vi "Simulator Tool Loop Dialog.vi"(1 "Tool Sim W1":u16, 2 "Tool Sim  W2":u16, 11 "error in (no error)":errorcluster) -> ()   [LabVIEW 2011]
uses:
  Measurments Handling/Status Digitalish.ctl
  Measurments Handling/Common/Variable List Common Analog.ctl
  Tool/Variable List Tool Analog.ctl
  Measurments Handling/Common/Variable List Common Digital.ctl
  Tool/Variable List Tool Digital.ctl
  Modem Status/Variable List Modem Status Analog.ctl
  Modem Status/Variable List Modem Status Digital.ctl
  Tool simulator data.ctl
  emi Lib/System 01/0 - General/App/Loop control 2/Private/_emi_SMLoop Control Single.vi
  emi Lib/System 01/0 - General/App/Loop control 2/Private/_emi_ SMLoop start condition.vi
  emi Lib/System 01/0 - General/App/Loop control 2/Private/_emi_ SMLoop Error Check.vi
  emi Lib/Basic/0 - General/Error/emi_Is Error.vi
  emi Lib/System 01/0 - General/App/Loop control 2/Private/_emi_SMLoop Register new.vi
  emi Lib/System 01/0 - General/S&E reporting/emi_Send S&E Error message.vi
  emi Lib/Basic/0 - General/Error/emi_ Is Error state.vi
  emi Lib/System 01/0 - General/emi_Read System ID.vi
  emi Lib/System 01/0 - General/App/Loop control/Private/_emi_GFV Loop Running.vi
  emi Lib/System 01/0 - General/App/Loop control 2/Private/_emi_ SMLoop Restart Counter.vi
  emi Lib/System 01/0 - General/App/Loop control/Private/_emi_GFV stop a loop so it can reset.vi
  emi Lib/System 01/0 - General/App/Loop control 2/Private/_emi_ SMLoop Restart.vi
  emi Lib/System 01/0 - General/App/Loop control/Private/_emi_GFV Loop Linking.vi
  emi Lib/System 01/0 - General/App/Loop control/Private/_emi_GFV Loop Enable.vi
  emi Lib/System 01/0 - General/App/Private/_emi_GFV App Close.vi
  emi Lib/System 01/0 - General/Private/_emi_GFV System ID.vi
  emi Lib/System 01/0 - General/S&E reporting/Private/_emi_S&E Q Generator.vi
  <vilib>/Utility/VariantDataType/GetNumericInfo.vi
  emi Lib/System 01/0 - General/Debug/Private/_emi_GFV Debug Disp.vi
panel:
  in  "Modem Status Digital Data":cluster{"Channel Name":string, "Status in":T1}[](array[cluster])
  in  "Modem Status Analog Data":T2(array[cluster]) {"Value" scale=0.0..100.0}
  in  "Tool Digital Data":cluster{"Channel Name":string, "Status in":T1}[](array[cluster])
  in  "PCP Digital Data":cluster{"Channel Name":string, "Status in":T1}[](array[cluster])
  in  "Loop timer - increase to create timeout":u32=250
  in  "PCP Simulator Data":T2(array[cluster]) {"Value" scale=0.0..100.0}
  in  "Simulator Data":T2(array[cluster]) {"Value" scale=0.0..200.0}
  # "Modem Status Data"
  # "PCP Data"
  # "Limited Tool simulator for GUI testing.\n\nNOTE: No tool behavior or properties should be infered absed on this simulator\ncapability. All tool capability and propertied information should go via propper\nproject channels."
  # "TOOL DATA"
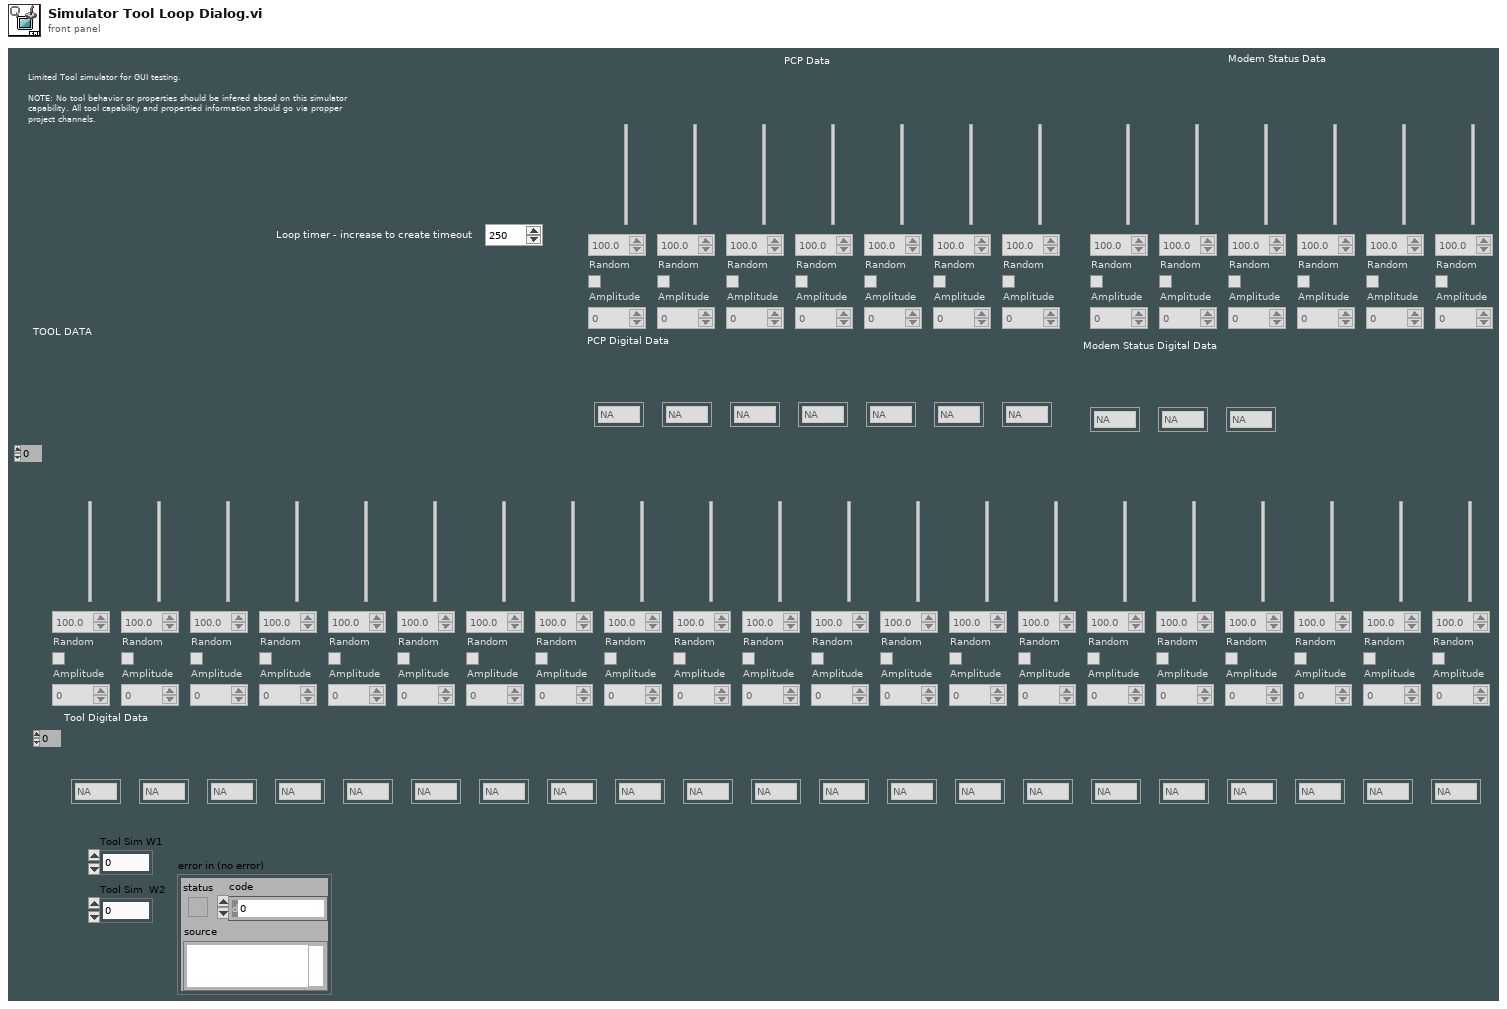
[diagram p1: front panel]
types:
  T1 = typedef "Status Digitalish.ctl" = enum16{"NA", "False", "True"}
  T2 = cluster{"Channel Name":string, "Value":dbl, "Random":bool, "Amplitude":dbl}[]
  T3 = typedef "Variable List Modem Status Digital.ctl" = enum16{"TMU_LINK_STATUS"}
  T4 = typedef "Variable List Modem Status Analog.ctl" = enum16{"TS_Signal_Quality", "TS_PCB_Temp", "TS_Gain", "DH_Signal_Quality", "DH_PCB_Temp", "DH_Gain", "Link_Status"}
  T5 = cluster{"Channel Name":string, "Value":dbl, "Random":bool, "Amplitude":dbl}
  T6 = typedef "Variable List Tool Digital.ctl" = enum16{"Tool Error Controller", "Tool Stopped Controller", "Tool Relay 1", "Tool Relay 2", "Tool Both Relays", "Tool node Pressure 1", "Tool Error Pressure 1", "Tool Stopped Pressure 1", "Tool node Pressure 2", "Tool Error Pressure 2", "Tool Stopped Pressure 2", "Tool node Solenoid", "Tool Error Solenoid", "Tool Stopped Solenoid", "Tool Solenoid 1", "Tool Solenoid 2", "Tool Solenoid 3", "Tool node PSU", "Tool Error PSU", "Tool Stopped PSU", "Upper Tension Sub", "Tool Error Upper Tension Sub", "Tool Stopped Upper Tension Sub", "Lower Tension Sub", "Tool Error Lower Tension Sub", "Tool Stopped Lower Tension Sub", "Stroke Target seeking", "Stroke Moving Out", "Stroke Moving Inn", "Stroke valves set for Out", "Stroke valves set for In", "Stroke In (force)", "Stroke Out (force)", "Stroke Force decreasing(in)", "Stroke Force decreasing(out)", "Stroke Force change not correct", "Stroke SLIPS established P1", "Stroke SLIPS established P2", "Stroke SLIPS established", "Stroke Pressure Monitor Ongoing", "Stroke Pressure Monitor Ending ", "Tool Stroke enable Valve", "Tool Stroke direction Valve", "Tool Anchor Valve", "Stroker Var19 - Reserved", "Stroker Var20 - Reserved", "Stroker Var21 - Reserved", "Stroker Var22 - Reserved", "Stroker Var23 - Reserved", "Stroker Var24 - Reserved", "Tractor Var1 - Reserved", "Tractor Var2 - Reserved", "Tractor Var3 - Reserved", "Tractor Var4 - Reserved", "Tractor Var5 - Reserved", "Tractor Var6 - Reserved", "Tractor Var7 - Reserved", "Tractor Var8 - Reserved", "Oil filling mode", "Mill Bit Direction", "Position control", "Anchor", "Driller Var5 - Reserved", "Driller Var6 - Reserved", "Driller Var7 - Reserved", "Driller Var8 - Reserved"}
  T7 = typedef "Variable List Common Digital.ctl" = enum16{"PCP Connected", "PCP PC Control", "HV PSU connected", "HV PSU HV Active", "Modem Connected", "Tool Connected", "CanBus interface"}
  T8 = typedef "Variable List Tool Analog.ctl" = enum16{"Tool Max Temperature", "Tool (Controller) Temperature", "Tool Supply Voltage", "Tool (Controller) Current", "Tool Acceleration X", "Tool Acceleration Y", "Tool Acceleration Z", "Tool Acceleration Sum", "Tool Inclination", "Tool Rotation", "Tool GP Sensor 1", "Tool GP Sensor 2", "Tool (Pressure 1) Temperature", "Tool Pressure 1 RAW", "Tool (Pressure 2) Temperature", "Tool Pressure 2 RAW", "Tool (Solenoid) Temperature", "Tool Solenoid Position", "PSU Temp", "Head Voltage", "PSU Main Voltage out", "PSU Main Current out", "Upper Tension Sub Temp", "Tool Upper Tension Sub Raw", "Lower Tension Sub Temp", "Tool Lower Tension Sub Raw", "Tool Var27 - Reserved", "Tool Var28 - Reserved", "Tool Var29 - Reserved", "Tool Var30 - Reserved", "Stroke Extension", "Stroke In Force", "Stroke Out Force", "Stroke Force", "Stroker Pressure 1", "Stroker Pressure 2", "Stroker Upper Tension Sub", "Stroker Lower Tension Sub", "Stroker Var09 - Reserved", "Stroker Var10 - Reserved", "Tractor Upper Tension Sub", "Tractor Lower Tension Sub", "Tractor Var03 - Reserved", "Tractor Var04 - Reserved", "Tool Temperature sensor", "Tool Motor Voltage", "Tool Motor Current", "Tool Motor Torque", "Tool weight on bit", "Tool Motor RPM"}
  T9 = typedef "Variable List Common Analog.ctl" = enum16{"HVPSU Head Voltage", "HVPSU TS Voltage", "HVPSU Current", "PCP Cable Resistance", "Winch Depth", "Winch Line Speed", "Winch Wire Tension"}
  T10 = typedef "Tool simulator data.ctl" = cluster{"Analog Values":dbl[], "Digital Values":T1[]}
  T11 = typedef "_emi_ SMLoop sates.ctl" = enum16{"Init", "Standby", "Start", "Normal Operation", "Stop", "Error Handling", "End", "Post"}
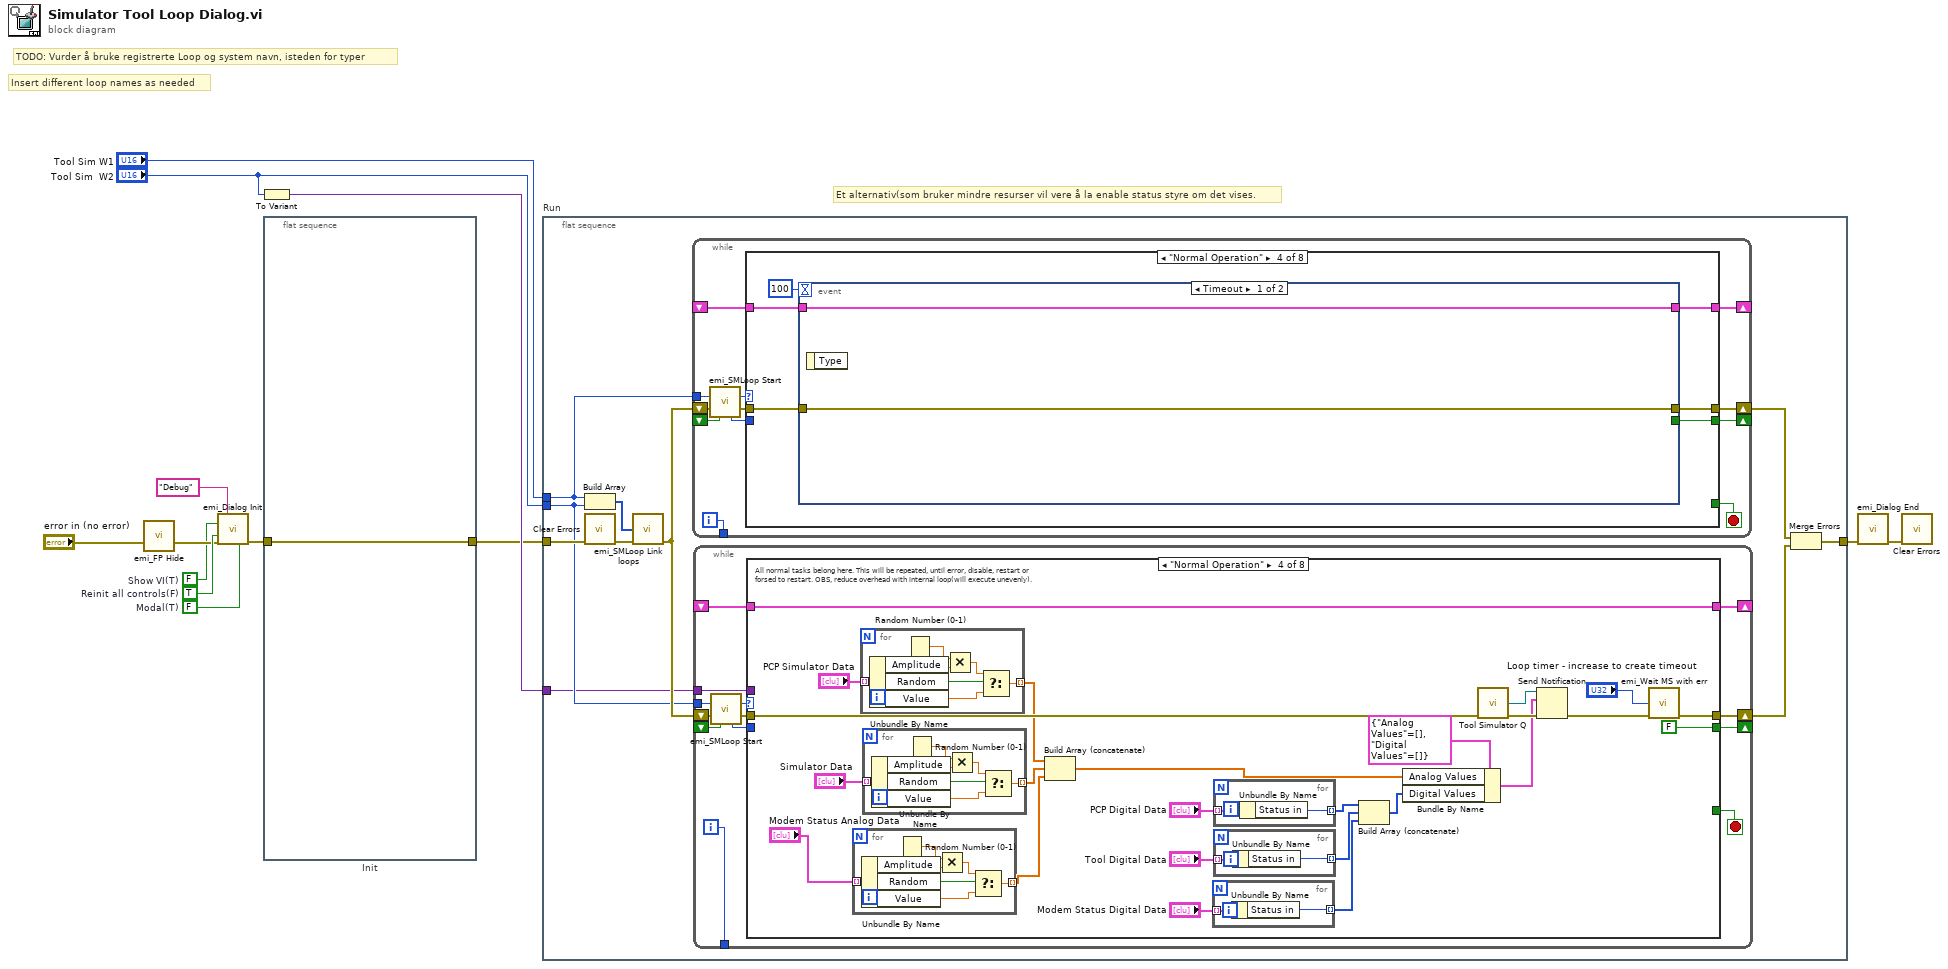
[diagram p0: block diagram]
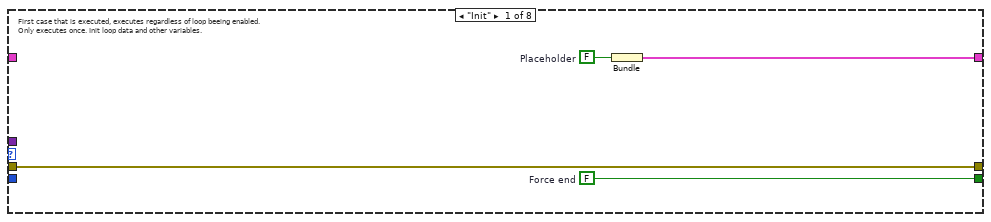
[diagram p2: hidden frame]
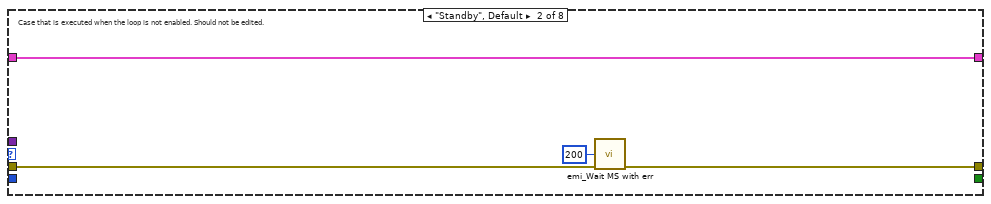
[diagram p3: hidden frame]
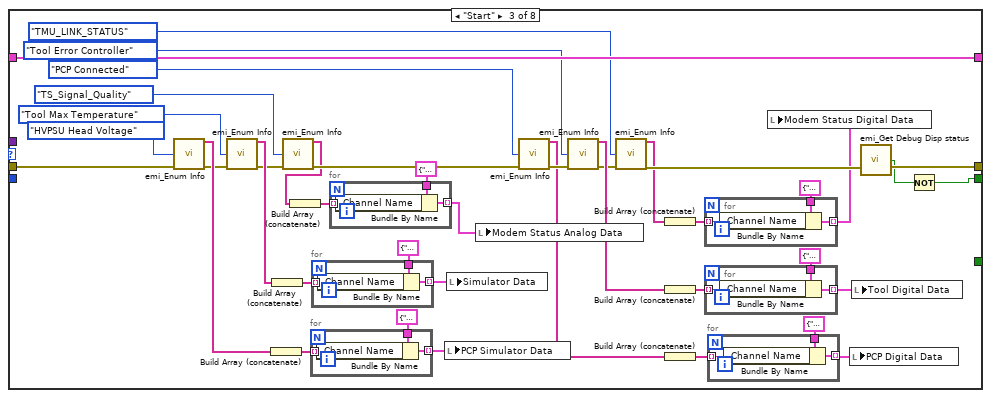
[diagram p4: hidden frame]
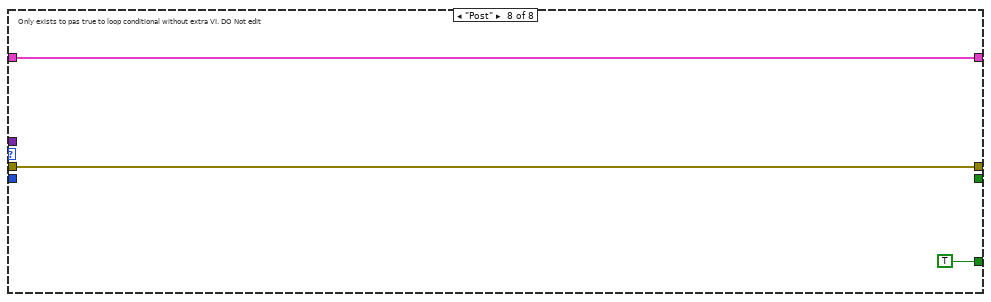
[diagram p8: hidden frame]
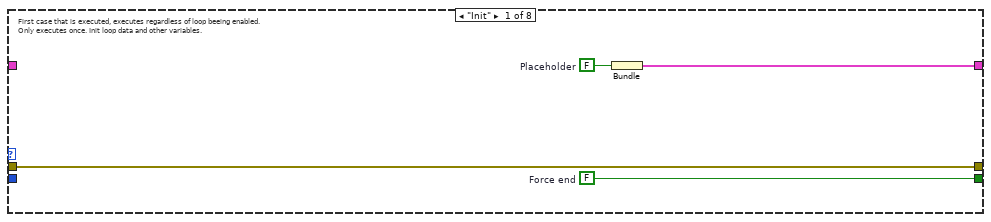
[diagram p9: hidden frame]
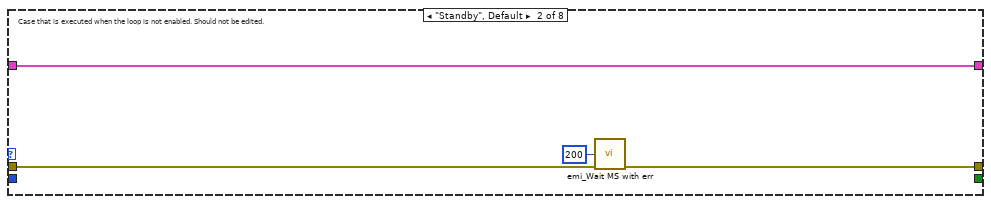
[diagram p10: hidden frame]
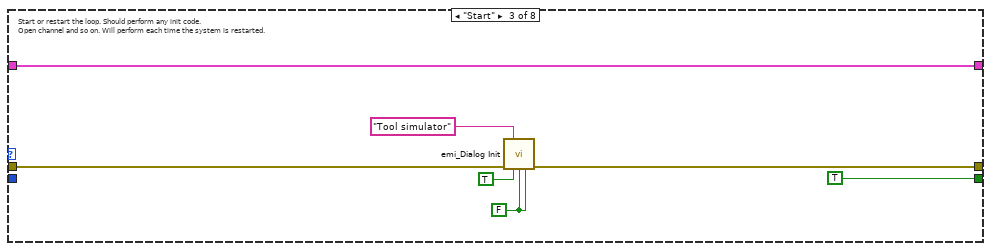
[diagram p11: hidden frame]
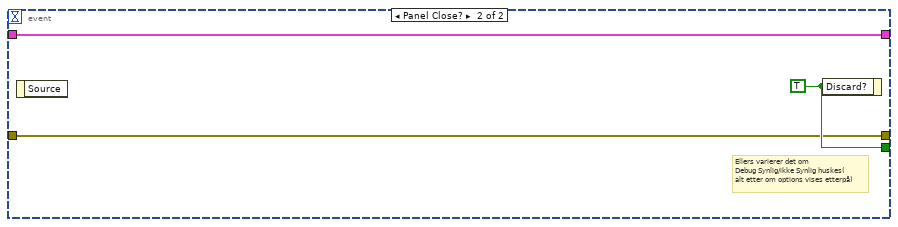
[diagram p12: hidden frame]
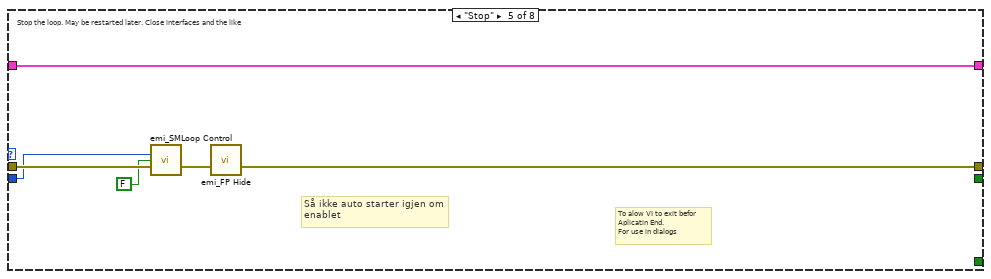
[diagram p13: hidden frame]
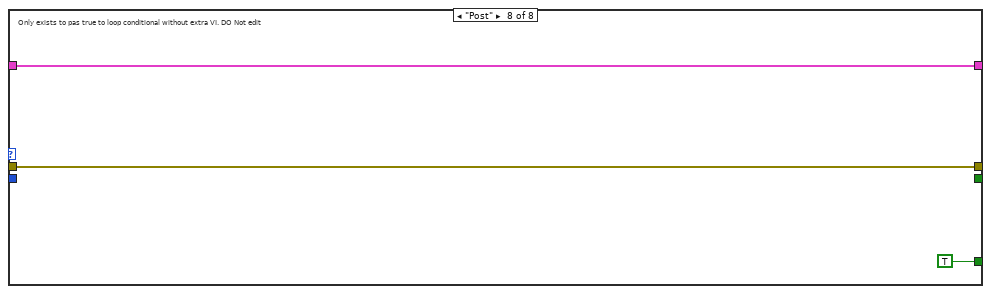
[diagram p16: hidden frame]
diagram:
  w8 = FALSE  # Show VI(T)
  w11 = TRUE  # Reinit all controls(F)
  w12 = FALSE  # Modal(T)
  # "Et alternativ(som bruker mindre resurser vil vere å la enable status styre om det vises."
  # "TODO: Vurder å bruke registrerte Loop og system navn, isteden for typer"
  # "Insert different loop names as needed"
  n1 = call "emi_FP Hide.vi"("error in (no error)"="error in (no error)") -> ("error out"=w10:errorcluster)  [unwired: 13 in, 1 out]
  n2 = call "emi_Dialog Init.vi"("Header String(\"\")"="Debug" ("Header String(\"\")"), "Show VI(T)"=w8, "Reinit all controls(F)"=w11, "error in"=w10, "Modal(T)"=w12) -> ("error out"=w9:errorcluster)  [unwired: 10 in]
  n3 = To Variant(anything="Tool Sim  W2") -> (Variant=w6:variant)
  n4 = flat-sequence "Init" {
    tunnel: [w14] -> w4
    tunnel: w9 -> [w14]
    frame #0 {
    }
  }
  n5 = flat-sequence "Run" {
    tunnel: w4 -> [w24]
    tunnel: [w21] -> w7
    tunnel: "Tool Sim W1" -> [w18]
    tunnel: "Tool Sim  W2" -> [w17]
    tunnel: w6 -> [w15]
    frame #0 {
      n6 = Build Array(w18, w17) -> (w16:u16[])
      n7 = call <vilib>:"Clear Errors.vi"("error in (no error)"=w24) -> ("error out"=w20:errorcluster)  [unwired: 6 in]
      n8 = call "emi_SMLoop Link loops.vi"("Loop IDS"=w16, "error in (no error)"=w20) -> ("error out"=w19:errorcluster)  [unwired: 13 in]
      n9 = while {
        shift-right: [w176] -> _
        shift-left: _ -> [w172]
        shift-right: [w174] -> w23
        shift-left: w19 -> [w170]
        tunnel: [w173] -> _
        shift-right: [w171] -> _
        shift-left: _ -> [w166]
        tunnel: w18 -> [w167]
        i -> [w173]
        stop <- w175 stop-if-true
        n10 = call "emi_SMLoop Start.vi"("Loop ID"=w167, "error in (no error)"=w170, "Force Stop(F)"=w166) -> ("Loop command"=w168:T11, "error out"=w169:errorcluster, "Loop ID out"=w165:i32)  [unwired: 10 in]
        n11 = case shown="\"Normal Operation\"" w168 {
          tunnel: [w179 w181 w191 w195 w208 w210 w211 w214] -> w176
          tunnel: [_ _ _ _ _ _ _ TRUE] -> w175
          tunnel: w169 -> [w180 w183 w186 w197 w207 w209 w212 w215]
          tunnel: [w180 w182 w190 w196 w204 w209 w212 w215] -> w174
          tunnel: w172 -> [_ w181 w191 w194 w208 w210 w211 w214]
          tunnel: [w177 _ TRUE ("Discard?") w193 _ _ _ _] -> w171
          tunnel: w165 -> [_ _ _ _ w206 _ _ _]
          frame "Init" {
            w177 = FALSE  # Force end
            w178 = FALSE  # Placeholder
            # "First case that is executed, executes regardless of loop beeing enabled.\nOnly executes once. Init loop data and other variables."
            n12 = Bundle("Placeholder"=w178) -> (w179:cluster{"Placeholder":bool})  [unwired: 1 in]
          }
          frame "Standby", Default {
            # "Case that is executed when the loop is not enabled. Should not be edited."
            n13 = call "emi_Wait MS with err.vi"("milliseconds to wait(0)"=u32 200, "error in (no error)"=w183) -> ("error out"=w182:errorcluster)  [unwired: 13 in]
          }
          frame "Start" {
            w185 = FALSE ("Set BG Color(T)")
            # "Start or restart the loop. Should perform any init code. \nOpen channel and so on. Will perform each time the system is restarted."
            n14 = call "emi_Dialog Init.vi"("Header String(\"\")"="Tool simulator" ("Header String(\"\")"), "error in"=w186, "Center in bottom FP(T)"=TRUE, "Set BG Color(T)"=w185, "Modal(T)"=w185) -> ("error out"=w190:errorcluster)  [unwired: 10 in]
          }
          frame "Normal Operation" {
            n15 = event shown="[0] Timeout" {
              selector: _ -> [_ _]
              dyn-events: _ -> [_ _]
              timeout: 100 -> [_ _]
              tunnel: w197 -> [w198 w200]
              tunnel: w194 -> [w199 w202]
              tunnel: [w199 w202] -> w195
              tunnel: [w198 w200] -> w196
              tunnel: [_ w201] -> w193
              event Timeout {
                n16 = event-data() -> ()  [unwired: 1 in, 1 out]
              }
              event Panel Close? {
                w201 = TRUE ("Discard?")
                # "Ellers varierer det om \nDebug Synlig/ikke Synlig huskes(\nalt etter om options vises etterpå)"
                n17 = event-data() -> ()  [unwired: 1 in, 1 out]
                n18 = event-data("Discard?"=w201) -> ()  [unwired: 1 in, 1 out]
              }
            }
          }
          frame "Stop" {
            # "Så ikke auto starter igjen om enablet"
            # "To alow VI to exit befor \nAplicatin End.\nFor use in dialogs"
            # "Stop the loop. May be restarted later. Close interfaces and the like"
            n19 = call-poly "emi_SMLoop Control.vi"("Loop ID in"=w206, "Enable"=FALSE, "error in (no error)"=w207) -> ("error out"=w205:errorcluster)  [unwired: 11 in, 1 out]
            n20 = call "emi_FP Hide.vi"("error in (no error)"=w205) -> ("error out"=w204:errorcluster)  [unwired: 13 in, 1 out]
          }
          frame "Error Handling" {
            # "Loop automaticaly returns here after error is found. If error is cleared, \nLoop wil continue as normal(if was operative when error."
          }
          frame "End" {
            # "Only executes at application end has. Should performa any action the loop \nneeds to finnish. Executes only once."
          }
          frame "Post" {
            # "Only exists to pas true to loop conditional without extra VI. DO Not edit"
          }
        }
      }
      n21 = while {
        shift-right: [w37] -> _
        shift-left: _ -> [w33]
        shift-right: [w35] -> w22
        shift-left: w19 -> [w31]
        tunnel: [w34] -> _
        shift-right: [w32] -> _
        shift-left: _ -> [w27]
        tunnel: w17 -> [w28]
        tunnel: w15 -> [w25]
        i -> [w34]
        stop <- w36 stop-if-true
        n22 = call "emi_SMLoop Start.vi"("Loop ID"=w28, "error in (no error)"=w31, "Force Stop(F)"=w27) -> ("Loop command"=w29:T11, "error out"=w30:errorcluster, "Loop ID out"=w26:i32)  [unwired: 10 in]
        n23 = case shown="\"Normal Operation\"" w29 {
          tunnel: [w41 w42 w86 w126 w156 w159 w160 w163] -> w37
          tunnel: [_ _ _ _ _ _ _ TRUE] -> w36
          tunnel: w30 -> [w38 w44 w82 w128 w157 w158 w161 w164]
          tunnel: [w38 w43 w85 w127 w157 w158 w161 w164] -> w35
          tunnel: w33 -> [_ w42 w86 w126 w156 w159 w160 w163]
          tunnel: [w39 _ w83 FALSE ("Force End") _ _ _ _] -> w32
          tunnel: w26 -> [_ _ _ _ _ _ _ _]
          tunnel: w25 -> [_ _ _ _ _ _ _ _]
          frame "Init" {
            w39 = FALSE  # Force end
            w40 = FALSE  # Placeholder
            # "First case that is executed, executes regardless of loop beeing enabled.\nOnly executes once. Init loop data and other variables."
            n24 = Bundle("Placeholder"=w40) -> (w41:cluster{"Placeholder":bool})  [unwired: 1 in]
          }
          frame "Standby", Default {
            # "Case that is executed when the loop is not enabled. Should not be edited."
            n25 = call "emi_Wait MS with err.vi"("milliseconds to wait(0)"=u32 200, "error in (no error)"=w44) -> ("error out"=w43:errorcluster)  [unwired: 13 in]
          }
          frame "Start" {
            n26 = call "emi_Enum Info.vi"("Enum"=Variable_List_Common_Analog."HVPSU Head Voltage" ("First part list"), "error in (no error)"=w82) -> ("Text Elements"=w80:string[], "error out"=w77:errorcluster)  [unwired: 10 in, 2 out]
            n27 = call "emi_Enum Info.vi"("Enum"=Variable_List_Tool_Analog."Tool Max Temperature" ("Variable ID"), "error in (no error)"=w77) -> ("Text Elements"=w72:string[], "error out"=w57:errorcluster)  [unwired: 10 in, 2 out]
            n28 = Build Array (concatenate)(w80) -> (w81:string[])
            n29 = Build Array (concatenate)(w72) -> (w73:string[])
            n30 = call "emi_Enum Info.vi"("Enum"=Variable_List_Modem_Status_Analog."TS_Signal_Quality" ("Variable ID"), "error in (no error)"=w57) -> ("Text Elements"=w50:string[], "error out"=w56:errorcluster)  [unwired: 10 in, 2 out]
            n31 = Build Array (concatenate)(w50) -> (w52:string[])
            n32 = for {
              tunnel: T5 {"Channel Name"="", "Value"=0.0, "Random"=FALSE, "Amplitude"=0.0} ("Simulator Data") -> [w104]
              tunnel: w81 -> [w103] mode=indexing
              tunnel: [w102] -> w79 mode=indexing
              n33 = Bundle By Name(cluster=w104, "Channel Name"=w103) -> (w102:T5)
            }
            n34 = for {
              tunnel: T5 {"Channel Name"="", "Value"=0.0, "Random"=FALSE, "Amplitude"=0.0} ("Simulator Data") -> [w101]
              tunnel: w73 -> [w100] mode=indexing
              tunnel: [w99] -> w71 mode=indexing
              n35 = Bundle By Name(cluster=w101, "Channel Name"=w100) -> (w99:T5)
            }
            n36 = for {
              tunnel: T5 {"Channel Name"="", "Value"=0.0, "Random"=FALSE, "Amplitude"=0.0} ("Simulator Data") -> [w89]
              tunnel: w52 -> [w88] mode=indexing
              tunnel: [w87] -> w46 mode=indexing
              n37 = Bundle By Name(cluster=w89, "Channel Name"=w88) -> (w87:T5)
            }
            n38 = local write "PCP Simulator Data"(w79) -> ()
            n39 = local write "Simulator Data"(w71) -> ()
            n40 = local write "Modem Status Analog Data"(w46) -> ()
            n41 = call "emi_Enum Info.vi"("Enum"=Variable_List_Common_Digital."PCP Connected" ("Action"), "error in (no error)"=w56) -> ("Text Elements"=w65:string[], "error out"=w70:errorcluster)  [unwired: 10 in, 2 out]
            n42 = call "emi_Enum Info.vi"("Enum"=Variable_List_Tool_Digital."Tool Error Controller", "error in (no error)"=w70) -> ("Text Elements"=w62:string[], "error out"=w59:errorcluster)  [unwired: 10 in, 2 out]
            n43 = call "emi_Enum Info.vi"("Enum"=Variable_List_Modem_Status_Digital."TMU_LINK_STATUS", "error in (no error)"=w59) -> ("Text Elements"=w53:string[], "error out"=w58:errorcluster)  [unwired: 10 in, 2 out]
            n44 = Build Array (concatenate)(w53) -> (w55:string[])
            n45 = Build Array (concatenate)(w62) -> (w63:string[])
            n46 = Build Array (concatenate)(w65) -> (w67:string[])
            n47 = for {
              tunnel: cluster{"Channel Name":string, "Status in":T1} {"Channel Name"="", "Status in"=enum."NA"} ("Simulator Data") -> [w92]
              tunnel: w55 -> [w91] mode=indexing
              tunnel: [w90] -> w47 mode=indexing
              n48 = Bundle By Name(cluster=w92, "Channel Name"=w91) -> (w90:cluster{"Channel Name":string, "Status in":T1})
            }
            n49 = for {
              tunnel: cluster{"Channel Name":string, "Status in":T1} {"Channel Name"="", "Status in"=enum."NA"} ("Simulator Data") -> [w95]
              tunnel: w63 -> [w94] mode=indexing
              tunnel: [w93] -> w60 mode=indexing
              n50 = Bundle By Name(cluster=w95, "Channel Name"=w94) -> (w93:cluster{"Channel Name":string, "Status in":T1})
            }
            n51 = for {
              tunnel: cluster{"Channel Name":string, "Status in":T1} {"Channel Name"="", "Status in"=enum."NA"} ("Simulator Data") -> [w98]
              tunnel: w67 -> [w97] mode=indexing
              tunnel: [w96] -> w61 mode=indexing
              n52 = Bundle By Name(cluster=w98, "Channel Name"=w97) -> (w96:cluster{"Channel Name":string, "Status in":T1})
            }
            n53 = local write "Modem Status Digital Data"(w47) -> ()
            n54 = local write "PCP Digital Data"(w61) -> ()
            n55 = local write "Tool Digital Data"(w60) -> ()
            n56 = call "emi_Get Debug Disp status.vi"("error in (no error)"=w58) -> ("Debug Disp"=w84:bool, "error out"=w85:errorcluster)  [unwired: 13 in]
            n57 = Not(x=w84) -> (.not. x?=w83:bool)
          }
          frame "Normal Operation" {
            # "All normal tasks belong here. This will be repeated, until error, disable, restart or\nforsed to restart. OBS, reduce overhead with internal loop(will execute unevenly)."
            n58 = for {
              tunnel: "Modem Status Analog Data" -> [w135] mode=indexing
              tunnel: [w129] -> w106 mode=indexing
              n59 = Unbundle By Name(w135) -> ("Amplitude"=w131:dbl, "Random"=w134:bool, "Value"=w133:dbl)
              n60 = Random Number (0-1)() -> (number: 0 to 1=w132:dbl)
              n61 = Multiply(x=w132, y=w131) -> (x*y=w130:dbl)
              n62 = Select(t=w130, s=w134, f=w133) -> (s? t:f=w129:dbl)
            }
            n63 = for {
              tunnel: "PCP Simulator Data" -> [w155] mode=indexing
              tunnel: [w149] -> w116 mode=indexing
              n64 = Unbundle By Name(w155) -> ("Amplitude"=w151:dbl, "Random"=w154:bool, "Value"=w153:dbl)
              n65 = Random Number (0-1)() -> (number: 0 to 1=w152:dbl)
              n66 = Multiply(x=w152, y=w151) -> (x*y=w150:dbl)
              n67 = Select(t=w150, s=w154, f=w153) -> (s? t:f=w149:dbl)
            }
            n68 = for {
              tunnel: "Simulator Data" -> [w148] mode=indexing
              tunnel: [w142] -> w114 mode=indexing
              n69 = Unbundle By Name(w148) -> ("Amplitude"=w144:dbl, "Random"=w147:bool, "Value"=w146:dbl)
              n70 = Random Number (0-1)() -> (number: 0 to 1=w145:dbl)
              n71 = Multiply(x=w145, y=w144) -> (x*y=w143:dbl)
              n72 = Select(t=w143, s=w147, f=w146) -> (s? t:f=w142:dbl)
            }
            n73 = Build Array (concatenate)(w116, w114, w106) -> (w117:dbl[])
            n74 = for {
              tunnel: "Modem Status Digital Data" -> [w137] mode=indexing
              tunnel: [w136] -> w107 mode=indexing
              n75 = Unbundle By Name(w137) -> ("Status in"=w136:T1)
            }
            n76 = for {
              tunnel: "PCP Digital Data" -> [w141] mode=indexing
              tunnel: [w140] -> w111 mode=indexing
              n77 = Unbundle By Name(w141) -> ("Status in"=w140:T1)
            }
            n78 = for {
              tunnel: "Tool Digital Data" -> [w139] mode=indexing
              tunnel: [w138] -> w109 mode=indexing
              n79 = Unbundle By Name(w139) -> ("Status in"=w138:T1)
            }
            n80 = Build Array (concatenate)(w111, w109, w107) -> (w110:T1[])
            n81 = Bundle By Name(cluster=T10 {"Analog Values"=[], "Digital Values"=[]} ("element"), "Analog Values"=w117, "Digital Values"=w110) -> (w120:T10)
            n82 = call "Tool Simulator Q.vi"("error in (no error)"=w128) -> ("Tool Data not"=w122:refnum<notifier>, "error out"=w123:errorcluster)  [unwired: 12 in, 1 out]
            n83 = Send Notification(notification=w120, notifier=w122, error in (no error)=w123) -> (error out=w119:errorcluster)  [unwired: 1 out]
            n84 = call "emi_Wait MS with err.vi"("milliseconds to wait(0)"="Loop timer - increase to create timeout", "error in (no error)"=w119) -> ("error out"=w127:errorcluster)  [unwired: 13 in]
          }
          frame "Stop" {
            # "To alow VI to exit befor \nAplicatin End.\nFor use in dialogs"
            # "Stop the loop. May be restarted later. Close interfaces and the like"
          }
          frame "Error Handling" {
            # "Loop automaticaly returns here after error is found. If error is cleared, \nLoop wil continue as normal(if was operative when error."
          }
          frame "End" {
            # "Only executes at application end has. Should performa any action the loop \nneeds to finnish. Executes only once."
          }
          frame "Post" {
            # "Only exists to pas true to loop conditional without extra VI. DO Not edit"
          }
        }
      }
      n85 = Merge Errors(w23, w22) -> (w21:errorcluster)
    }
  }
  n86 = call "emi_Dialog End.vi"("error in"=w7) -> ("error out"=w3:errorcluster)  [unwired: 14 in]
  n87 = call <vilib>:"Clear Errors.vi"("error in (no error)"=w3) -> ()  [unwired: 6 in, 1 out]
